vi "Redis_Example1.vi"() -> ()   [LabVIEW 2020]
doc: "This VI shows an example of the Redis in LabVIEW palette use.\n\nThe first and last VIs allow connection to the Redis DB, then \"HSET\" and \"HGET\" functions present a simple write and read data feature."
uses:
  SubVIs/Controls/redis-data.ctl
  Palette/Redis Commands/Hashes/HSET.vi
  Palette/Redis Commands/Hashes/HGET.vi
panel:
  out "error out":errorcluster
  out "Data":T1
  in  "Value":string
  in  "Field":string
  in  "Key":string
  in  "Host":string="localhost"
  in  "Port":u16=6379
  in  "error in":errorcluster
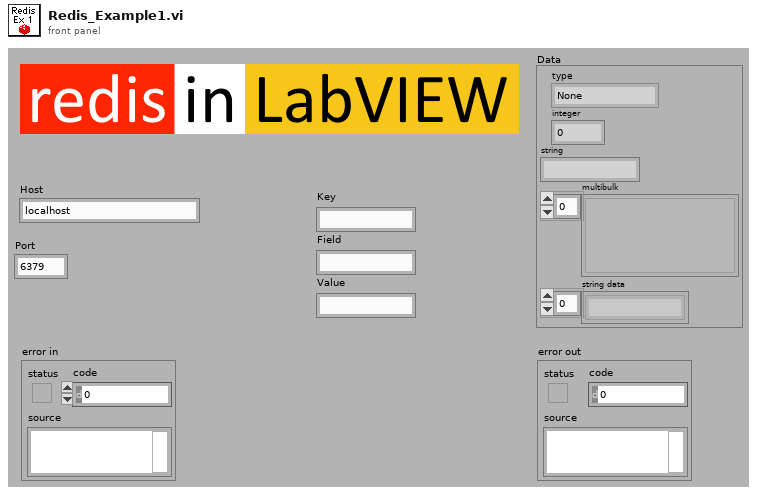
[diagram p1: front panel]
types:
  T1 = typedef "redis-data.ctl" = cluster{"type":enum16{"None", "Error", "Status", "Nil", "Integer", "String", "Multibulk"}, "integer":i64, "string":string, "multibulk":variant[], "string data":string[]}
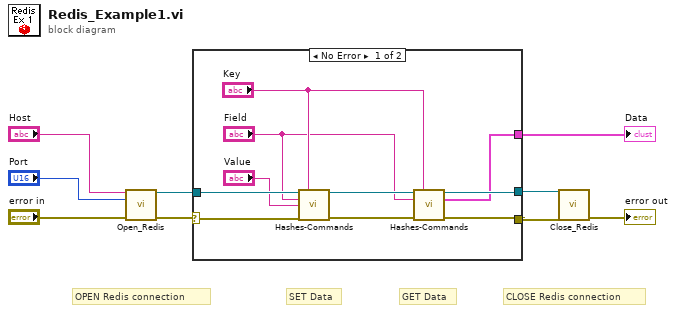
[diagram p0: block diagram]
diagram:
  # "CLOSE Redis connection"
  # "GET Data"
  # "SET Data"
  # "OPEN Redis connection"
  n1 = call "Open_Redis.vi"("Host"="Host", "Port"="Port", "error in"="error in") -> ("Refnum out"=w5:refnum<vi>, "error out"=w6:errorcluster)  [unwired: 10 in, 1 out]
  n2 = case shown="No Error" w6 {
    selector: w6 -> [w18 w20]
    tunnel: w5 -> [w19 w21]
    tunnel: [w12 w20] -> w3
    tunnel: [w11 w21] -> w4
    tunnel: [w10 _] -> w2
    frame No Error {
      n3 = call-poly "Hashes-Commands.vi"("refnum in"=w19, "Key"="Key", "Field"="Field", "Value"="Value", "error in"=w18) -> ("refnum out"=w15:refnum<vi>, "error out"=w16:errorcluster)  [unwired: 8 in, 1 out]
      n4 = call-poly "Hashes-Commands.vi"("refnum in"=w15, "Key"="Key", "Field"="Field", "error in"=w16) -> ("refnum out"=w11:refnum<vi>, "Data"=w10:T1, "error out"=w12:errorcluster)  [unwired: 9 in]
    }
    frame Error {
    }
  }
  "Data" <- w2
  n5 = call "Close_Redis.vi"("Refnum in"=w4, "error in"=w3) -> ("error out"=→"error out":errorcluster)  [unwired: 10 in, 3 out]
